vi "Image Processing with Vision Assistant on 1473R (FPGA).vi"() -> ()   [LabVIEW 2014]
doc: "This is the FPGA VI for the 1-Tap 8-Bit Camera with Centroid example. This example demonstrates how to perform image processing operations on the FPGA in real time. This example performs an image thresholding operation, which can be controlled via the host VI, followed by a centroid computation. The processed images and centroid coordinates are then transfered to the host, using DMA, so that they can be displayed.\n\nAdditionally, the example demonstrates the serial server, which allows third-party camera configuration utilities to communicate with the camera using the Camera Link serial interface while this VI is running."
uses:
  SubVIs/CL Signal Mapping.ctl
  SubVIs/CL Configuration.ctl
  <vilib>/visionFPGA/Controls/IMAQ FPGA Image Size.ctl
  <vilib>/Platform/TimedLoop/XDataNode/timing_clust.ctl
  <vilib>/Platform/TimedLoop/XDataNode/nitl_modes.ctl
  <vilib>/Platform/TimedLoop/XDataNode/wakeup.ctl
  <vilib>/rvi/Emulation/niFpgaGetClockAttributes.vi
  <vilib>/rvi/Emulation/niFpgaSctlEmulationGetInTimedLoop.vi
  <vilib>/rvi/Emulation/niFpgaEmulationReportErrorSimple.vi
  <vilib>/rvi/Emulation/niFpgaProcessEmulError.vi
  <vilib>/rvi/Emulation/niFpgaCriticalErrorInLSC.vi
  <vilib>/rvi/eio/common/nirviEmuTemplateMethod_errors.vi
  SubVIs/CL Data to Pixels/1 Tap 8-Bit.vi
  <vilib>/rvi/DataTransferAndStorage/Container/Common/niFpgaContainerGetUniqueNameForEmu.vi
  <vilib>/rvi/DataTransferAndStorage/Container/Common/niFpgaContainerSetEmuInfo.vi
  <vilib>/rvi/eio/common/nirviEmuReportErrorAndStop.vi
  <vilib>/visionFPGA/Basics/FIFO to Pixel Bus/IMAQ FPGA FIFO to Pixel Bus U8x1.vi
  <vilib>/visionFPGA/Basics/Pixel Bus to FIFO/IMAQ FPGA Pixel Bus to FIFO U8x1.vi
  <vilib>/rvi/DataTransferAndStorage/Container/Common/niFpgaContainerExecOnDevCompGetState.vi
  <vilib>/rvi/Emulation/niFpgaEmulationIsFPGAContextNoSignature.vi
  <vilib>/rvi/errors/niFpgaSetErrorForExecOnDevCompSimple.vi
  <vilib>/rvi/FIFO/Fifo_Resource/nirvififoEmulationSetSize.vi
  <vilib>/rvi/FIFO/Fifo_Resource/nirviFifoEmulationQueueMgr.vi
  <instcachedir>/0/nirviFifoEmulationQueueMgr_E5CAEC123FF24DC58D834DCA3CDAA9B5.lvgen/nirviFifoEmulationQueueMgr_E5CAEC123FF24DC58D834DCA3CDAA9B5_003.vi
  <vilib>/rvi/FIFO/Fifo_Resource/nirvififoEmulationDetermineInputValidOut.vi
  <vilib>/rvi/FIFO/Fifo_Resource/nirvififoEmulationCreateLock.vi
  <vilib>/rvi/FIFO/Fifo_Resource/nirvififoEmulationObtainLock.vi
  <vilib>/rvi/FIFO/Fifo_Resource/nirvififoEmulationReleaseLock.vi
  <vilib>/rvi/occurrence/nirviWaitOnOccurrenceBase.vi
  <vilib>/rvi/errors/nirviReportUnexpectedCaseInternalError.vi
  <vilib>/rvi/errors/nirviReportUnexpectedCaseInternalError (U32).vi
  <vilib>/rvi/interface/RandomDataEmulation/niFpgaRandomDataHandleErrors.vi
  <vilib>/eio/EIONode/EIONode.xnode
  <vilib>/Platform/TimedLoop/XDataNode/XDataNode.xnode
  <vilib>/rvi/LocalResourceManager/LocalResourceManager.xnode
  <vilib>/rvi/DataTransferAndStorage/Container/XNode/niFpgaContainer.xnode
  <vilib>/rvi/FIFO/Fifo_Resource/niFpgaFifoEmulationRefIn.vi
  <vilib>/Platform/TimedLoop/XDataNode/XDNodeRunTimeDep.lvlib
  <vilib>/visionFPGA/NI_VDM_FPGA_Basics.lvlib
panel:
  in  "Image Size":T1
  in  "CL Config.Configuration":T2
  in  "CL Config.Signal Mapping":T3
  in  "CL Config.Line Scan":bool
  in  "CL Config.DVAL Active High":bool=TRUE
  in  "CL Config.LVAL Active High":bool=TRUE
  in  "CL Config.FVAL Active High":bool=TRUE
  in  "CL Config.Spare Active High":bool=TRUE
  in  "Acq Control.Line Scan Height":u32
  in  "Acq Control.Frames To Acq":u32
  in  "Acq Control.Acquire":bool
  in  "Acq Control.Cancel Acq":bool
  in  "Acq Control.Ignore DVAL":bool
  in  "Acq Control.Initialize":bool
  out "Acq Status.Acq In Progress":bool
  out "Acq Status.Clocks Per Line":u32
  out "Acq Status.Frames Acq'd":u32
  out "Acq Status.Lines Per Frame":u32
  out "Acq Status.Acquisition Overflow":bool
  out "Acq Status.Initialized":bool
  in  "UART.Baud Rate":u8
  in  "UART.Transmit":bool
  in  "UART.Tx Data":u8[](array[numeric])=[0, 0, 0, 0, 0, 0, 0, 0, 0, 0] format="%02x"
  in  "UART.Set Baud Rate":bool
  in  "UART.Byte Mode":bool=TRUE
  out "UART.Rx Ready":bool
  out "UART.Break Indicator":bool
  out "UART.Framing Error":bool
  out "UART.Overrun Error":bool
  out "UART.Tx Ready":bool
  out "UART.Rx Data":u8 format="%02x"
  in  "UART.Receive":bool
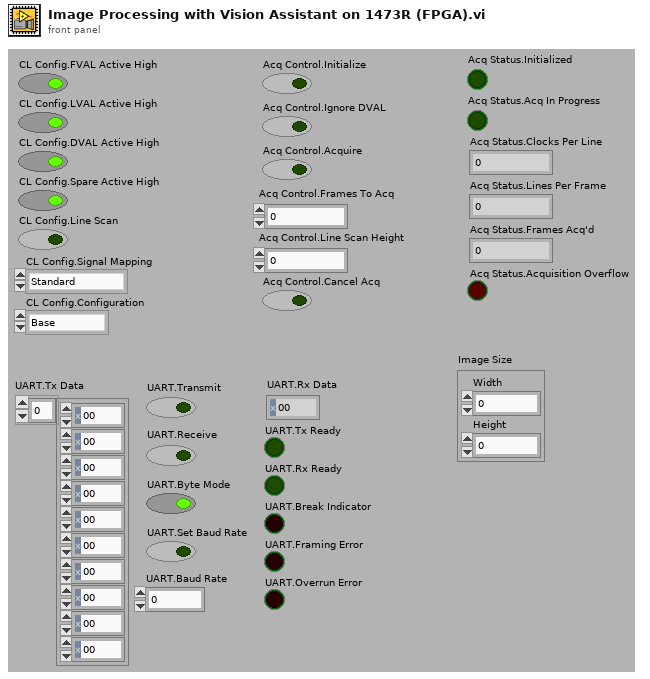
[diagram p1: front panel]
types:
  T1 = typedef "IMAQ FPGA Image Size.ctl" = cluster{"Width":u32, "Height":u32}
  T2 = typedef "CL Configuration.ctl" = enum8{"Base", "Medium", "Full"}
  T3 = typedef "CL Signal Mapping.ctl" = enum8{"Standard", "Basler 10-tap", "Vosskühler 10-tap"}
  T4 = typedef "XDNodeRunTimeDep.lvlib/timing_clust.ctl" = cluster{"Expected End [f-1]":u64, "Actual End [f-1]":u64, "Finished Late? [f-1]":bool, "Expected End [i-1]":u64, "Actual End [i-1]":u64, "Finished Late? [i-1]":bool, "Expected Start [i]":u64, "Actual Start [i]":u64, "Expected Start [f]":u64, "Actual Start [f]":u64, "Source Name":string, "Structure Name":string, "Period":i64, "Deadline":i64, "Offset":i64, "Start":i64, "Priority":i32, "Timeout":i32, "Mode":T5, "Wakeup Reason":T6, "Error":errorcluster, "Source Type":string, "Secondary Source Type":string, "Global End Time":u64, "Global Start Time":u64, "Frame Duration":u64, "Iteration Duration":u64, "Assigned CPU":i32, "I/O Scan Engine Mode":u32}
  T5 = typedef "XDNodeRunTimeDep.lvlib/nitl_modes.ctl" = enum32{"No Change", "Process missed periods, maintain original phase", "Discard missed periods, maintain original phase", "Process missed periods, ignore original phase", "Discard missed periods, ignore original phase"}
  T6 = typedef "XDNodeRunTimeDep.lvlib/wakeup.ctl" = enum32{"Normal", "Aborted", "Asynchronous wakeup", "Timing source error", "Timed loop error", "Timeout"}
  T7 = cluster{"Enables Valid":bool, "Frame Valid":bool, "Line Valid":bool, "Data Valid":bool}
  T8 = typedef "IMAQ FPGA Pixel Bus u8x1.ctl" = cluster{"Pixel Data":u8, "DV":bool, "EOL":bool, "EOI":bool, "Data Type":enum16{"U8 x 1"}}
  T9 = cluster{"Tx Data":u8[], "Transmit":bool, "Receive":bool, "Byte Mode":bool, "Set Baud Rate":bool, "Baud Rate":u8}
  T10 = cluster{"Rx Data":u8, "Turn Off Transmit":bool, "Turn Off Receive":bool, "Turn Off Set Baud Rate":bool, "Tx Ready":bool, "Rx Ready":bool, "Break Indicator":bool, "Framing Error":bool, "Overrun Error":bool}
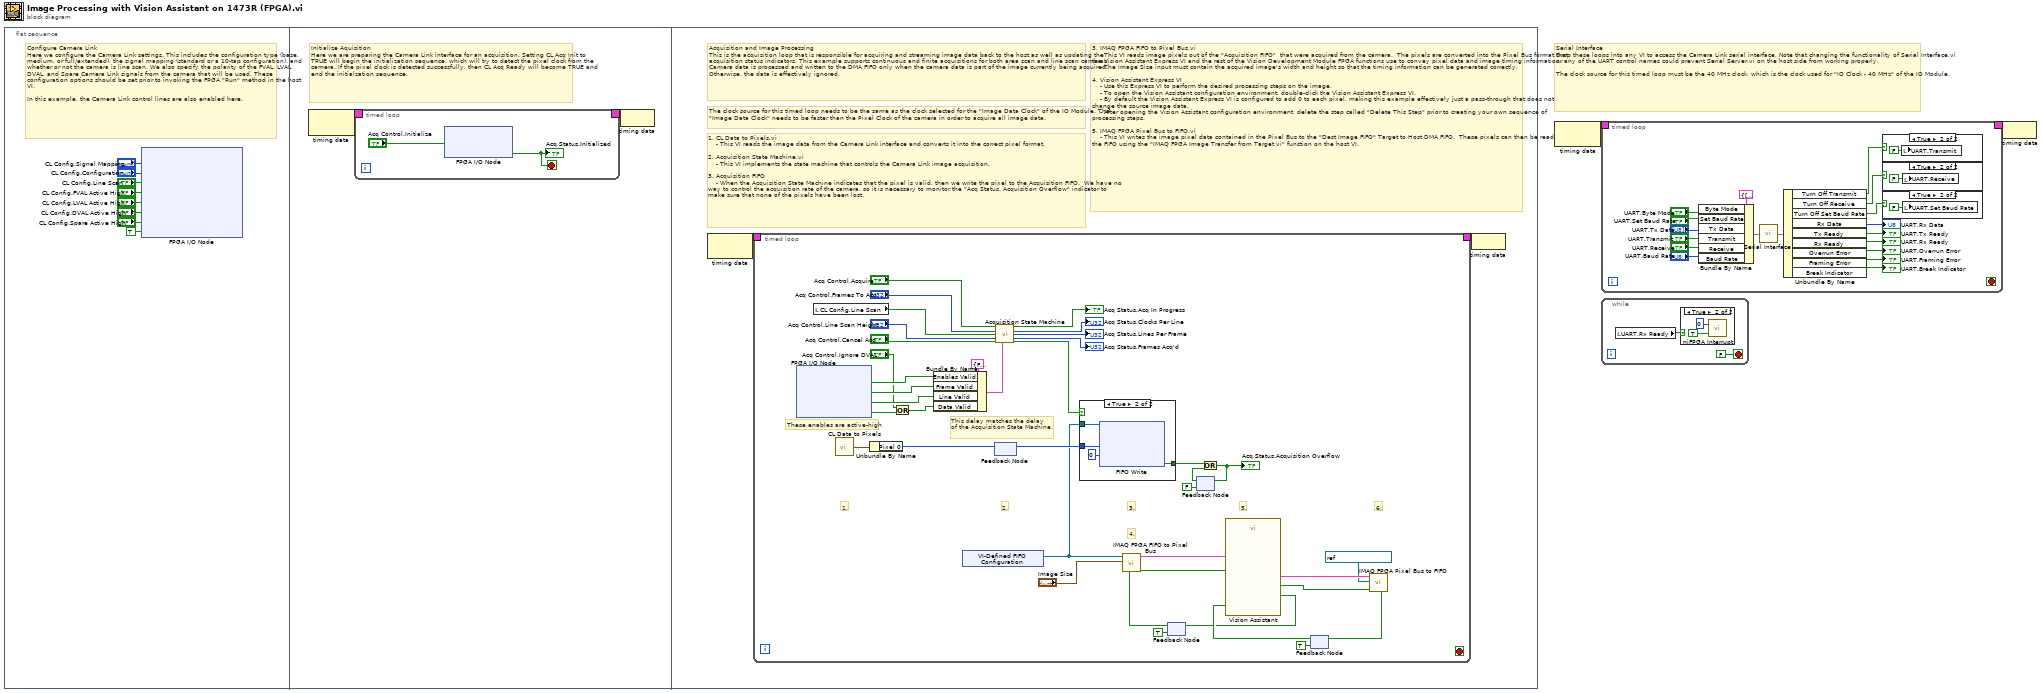
[diagram p0: block diagram]
diagram:
  # "Serial Interface\nDrop these loops into any VI to access the Camera Link serial interface. Note that changing the functionality of Serial Interface.vi or any of the UART control names could prevent Serial Server.vi on the host side from working properly.\n\nThe clock source for this timed loop must be the 40 MHz clock, which is the clock used for \"IO Clock - 40 MHz\" of the IO Module."
  n1 = flat-sequence {
    frame #0 {
      # "Configure Camera Link\nHere we configure the Camera Link settings. This includes the configuration type (base, medium, or full/extended), the signal mapping (standard or a 10-tap configuration), and whether or not the camera is line scan. We also specify the polarity of the FVAL, LVAL, DVAL, and Spare Camera Link signals from the camera that will be used. These configuration options should be set prior to invoking the FPGA \"Run\" method in the host VI.\n\nIn this example, the Camera Link control lines are also enabled here."
      n2 = xnode "FPGA I/O Node"("CL Set Signal Mapping"="CL Config.Signal Mapping", "CL Set Configuration"="CL Config.Configuration", "CL Set Line Scan"="CL Config.Line Scan", "CL Set FVAL Active High"="CL Config.FVAL Active High", "CL Set LVAL Active High"="CL Config.LVAL Active High", "CL Set DVAL Active High"="CL Config.DVAL Active High", "CL Set Spare Active High"="CL Config.Spare Active High", "CL Control Enable"=TRUE ("IO Module\\CL Control Enable")) -> ()  [unwired: 8 in, 8 out]
    }
    frame #1 {
      # "Initialize Aquisition\nHere we are preparing the Camera Link interface for an acquisition. Setting CL Acq Init to TRUE will begin the initialization sequence, which will try to detect the pixel clock from the camera. If the pixel clock is detected successfully, then CL Acq Ready will become TRUE and end the initialzation sequence."
      n3 = node-c288() -> (w12:T4)  [unwired: 1 out]
      n4 = timed-loop {
        timing: w12 -> [_]
        timing-out: [_] -> w11
        stop <- w13 stop-if-true
        n5 = xnode "FPGA I/O Node"("CL Acq Init"="Acq Control.Initialize") -> ("CL Acq Ready"=w13:bool)  [unwired: 2 in, 2 out]
        "Acq Status.Initialized" <- w13
      }
      n6 = node-c288(w11) -> ()
    }
    frame #2 {
      # "1. CL Data to Pixels.vi\n    - This VI reads the image data from the Camera Link interface and converts it into the correct pixel format.\n\n2. Acquisition State Machine.vi\n    - This VI implements the state machine that controls the Camera Link image acquisition.\n\n3. Acquisition FIFO\n    - When the Acquisition State Machine indicates that the pixel is valid, then we write the pixel to the Acquisition FIFO.  We have no way to control the acquisition rate of the camera, so it is necessary to monitor the \"Acq Status. Acquisition Overflow\" indicator to make sure that none of the pixels have been lost."
      # "3. IMAQ FPGA FIFO to Pixel Bus.vi\n    - This VI reads image pixels out of the \"Acquisition FIFO\"  that were acquired from the camera.  The pixels are converted into the Pixel Bus format that the Vision Assistant Express VI and the rest of the Vision Development Module FPGA functions use to convey pixel data and image timing information.\n    - The Image Size input must contain the acquired image's width and height so that the timing information can be generated correctly.\n\n4. Vision Assistant Express VI\n    - Use this Express VI to perform the desired processing steps on the image.\n    - To open the Vision Assistant configuration environment, double-click the Vision Assistant Express VI.\n    - By default the Vision Assistant Express VI is configured to add 0 to each pixel, making this example effectively just a pass-through that does not change the source image data.\n    - After opening the Vision Assistant configuration environment, delete the step called \"Delete This Step\" prior to creating your own sequence of processing steps.\n\n5. IMAQ FPGA Pixel Bus to FIFO.vi\n    - This VI writes the image pixel data contained in the Pixel Bus to the \"Dest Image FIFO\" Target to Host DMA FIFO.  These pixels can then be read out of the FIFO using the \"IMAQ FPGA Image Transfer from Target.vi\" function on the host VI."
      # "The clock source for this timed loop needs to be the same as the clock selected for the \"Image Data Clock\" of the IO Module. The \"Image Data Clock\" needs to be faster than the Pixel Clock of the camera in order to acquire all image data."
      # "Acquisition and Image Processing\nThis is the acquisition loop that is responsible for acquiring and streaming image data back to the host as well as updating the acquisition status indicators. This example supports continuous and finite acquisitions for both area scan and line scan cameras. Camera data is processed and written to the DMA FIFO only when the camera data is part of the image currently being acquired. Otherwise, the data is effectively ignored."
      n7 = node-c288() -> (w20:T4)  [unwired: 1 in]
      n8 = timed-loop {
        timing: w20 -> [_]
        timing-out: [_] -> w19
        stop <- _ stop-if-true
        # "2."
        # "6."
        # "1."
        # "5."
        # "4."
        # "3."
        # "These enables are active-high"
        # "This delay matches the delay\nof the Acquisition State Machine."
        n9 = xnode "FPGA I/O Node"() -> ("CL Output Valid"=w49:bool, "CL Frame Valid"=w48:bool, "CL Line Valid"=w47:bool, "CL Data Valid"=w44:bool)  [unwired: 4 in, 4 out]
        n10 = local read "CL Config.Line Scan"() -> (w41:bool)
        n11 = call-poly "CL Data to Pixels.vi"() -> ("Pixels"=w58:cluster{"Pixel 0":u8})  [unwired: 1 in]
        n12 = Unbundle By Name(w58) -> ("Pixel 0"=w57:u8)
        n13 = Or(x="Acq Control.Ignore DVAL", y=w44) -> (x .or. y?=w43:bool)
        n14 = Bundle By Name(cluster=T7 {"Enables Valid"=FALSE, "Frame Valid"=FALSE, "Line Valid"=FALSE, "Data Valid"=FALSE} ("Enables"), "Enables Valid"=w49, "Frame Valid"=w48, "Line Valid"=w47, "Data Valid"=w43) -> (w46:T7)
        n15 = xnode "VI-Defined FIFO Configuration"() -> ("FIFO Out"=w34:refnum<k21>)
        n16 = feedback-in #1(w57) -> ()
        n17 = feedback #1() -> (w36:u8)  [unwired: 1 in]
        n18 = call "Acquisition State Machine.vi"("Acquire"="Acq Control.Acquire", "Frames to Acquire"="Acq Control.Frames To Acq", "Line Scan"=w41, "Line Scan Height"="Acq Control.Line Scan Height", "Cancel Acq"="Acq Control.Cancel Acq", "Enables"=w46) -> ("Acq In Progress"=→"Acq Status.Acq In Progress":bool, "Num Clocks Per Line"=→"Acq Status.Clocks Per Line":u32, "Num Lines Per Frame"=→"Acq Status.Lines Per Frame":u32, "Num Frames Acq'd"=→"Acq Status.Frames Acq'd":u32, "Capture Cycle"=w35:bool)  [unwired: 4 in, 1 out]
        n19 = case shown="True" w35 {
          tunnel: w34 -> [_ w60]
          tunnel: w36 -> [_ w62]
          tunnel: [_ w61] -> w33
          frame False {
          }
          frame True {
            n20 = xnode "FIFO Write"("Element"=w62, "Timeout"=0, "FIFO In"=w60) -> ("Timed Out?"=w61:bool)  [unwired: 1 out]
          }
        }
        n21 = feedback #2(TRUE ("Ready for Input")) -> (w24:bool)
        n22 = call-poly <vilib>:"IMAQ FPGA FIFO to Pixel Bus.vi"("Ready For Output"=w24, "Image Size"="Image Size", "Source Image FIFO"=w34) -> ("Output Valid"=w30:bool, "Pixel Bus Out"=w31:T8)  [unwired: 6 in, 1 out]
        n23 = feedback #3(FALSE) -> (w38:bool)
        n24 = Or(x=w33, y=w38) -> (x .or. y?=w37:bool)
        "Acq Status.Acquisition Overflow" <- w37
        n25 = feedback-in #3(w37) -> ()
        n26 = feedback #4(TRUE ("Ready for Input")) -> (w26:bool)
        n27 = call "Vision Assistant"("Pixel Bus"=w31, "Input Valid"=w30, "Ready for Output"=w26) -> ("Pixel Bus Out"=w29:T8, "Output Valid"=w28:bool, "Ready for Input"=w25:bool)  [unwired: 22 in]
        n28 = feedback-in #2(w25) -> ()
        n29 = call-poly <vilib>:"IMAQ FPGA Pixel Bus to FIFO.vi"("Input Valid"=w28, "Destination Image FIFO"=refnum<k21> "Dest Image FIFO", "Pixel Bus In"=w29) -> ("Ready for Input"=w27:bool)  [unwired: 8 in]
        n30 = feedback-in #4(w27) -> ()
      }
      n31 = node-c288(w19) -> ()
    }
  }
  n32 = node-c288() -> (w2:T4)  [unwired: 1 out]
  n33 = timed-loop {
    timing: w2 -> [_]
    timing-out: [_] -> w1
    stop <- _ stop-if-true
    n34 = Bundle By Name(cluster=T9 {"Tx Data"=[0, 0, 0, 0, 0, 0, 0, 0, 0, 0], "Transmit"=FALSE, "Receive"=FALSE, "Byte Mode"=TRUE, "Set Baud Rate"=FALSE, "Baud Rate"=0} ("UART Inputs"), "Byte Mode"="UART.Byte Mode", "Set Baud Rate"="UART.Set Baud Rate", "Tx Data"="UART.Tx Data", "Transmit"="UART.Transmit", "Receive"="UART.Receive", "Baud Rate"="UART.Baud Rate") -> (w67:T9)
    n35 = call "Serial Interface.vi"("UART Inputs"=w67) -> ("UART Outputs"=w79:T10)
    n36 = Unbundle By Name(w79) -> ("Turn Off Transmit"=w72:bool, "Turn Off Receive"=w73:bool, "Turn Off Set Baud Rate"=w69:bool, "Rx Data"=→"UART.Rx Data":u8, "Tx Ready"=→"UART.Tx Ready":bool, "Rx Ready"=→"UART.Rx Ready":bool, "Overrun Error"=→"UART.Overrun Error":bool, "Framing Error"=→"UART.Framing Error":bool, "Break Indicator"=→"UART.Break Indicator":bool)
    n37 = case shown="True" w72 {
      frame False {
      }
      frame True {
        n38 = local write "UART.Transmit"(FALSE ("UART.Transmit")) -> ()
      }
    }
    n39 = case shown="True" w73 {
      frame False {
      }
      frame True {
        n40 = local write "UART.Receive"(FALSE ("UART.Receive")) -> ()
      }
    }
    n41 = case shown="True" w69 {
      frame False {
      }
      frame True {
        n42 = local write "UART.Set Baud Rate"(FALSE ("UART.Receive")) -> ()
      }
    }
  }
  n43 = while {
    stop <- FALSE stop-if-true
    n44 = local read "UART.Rx Ready"() -> (w91:bool)
    n45 = case shown="True" w91 {
      frame False {
      }
      frame True {
        n46 = call <vilib>:"niFPGA Interrupt.vi"("Wait Until Cleared (F)"=TRUE ("Wait Until Cleared"), "IRQ Number (0)"=u8 0 ("IRQ Number")) -> ()  [unwired: 1 in]
      }
    }
  }
  n47 = node-c288(w1) -> ()
